vi "Get Edge Mode.vi"(8 "error in (no error)":errorcluster, 11 "VISA resource name":refnum<visa-resource-name>) -> (0 "error out":errorcluster, 2 "Edge Mode":i32, 3 "VISA resource name out":refnum<visa-resource-name>)   [LabVIEW 2013, in "Fluke 5XXX Series Multicalibrators.lvlib"]
doc: "This VI returns the tunnel diode pulse drive setting in the Edge scope mode.\n\nNote:\n\nThis VI is available only for instrument models 5500A and 5520A with oscilloscope option SC600 (SC1100)."
uses:
  Fluke 5XXX Series Multicalibrators.lvlib
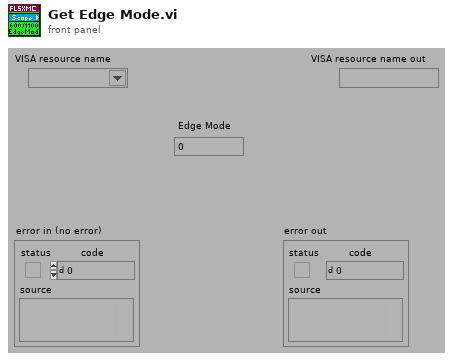
[diagram p1: front panel]
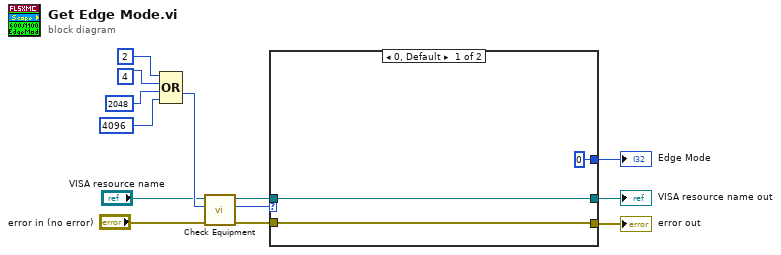
[diagram p0: block diagram]
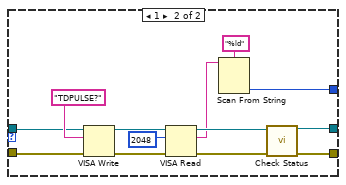
[diagram p2: hidden frame]
diagram:
  n1 = Compound Arithmetic op=OR(2 ("Numeric"), 4 ("Numeric"), 2048 ("Numeric"), 4096 ("Numeric")) -> (w10:i32)
  n2 = call "Check Equipment.vi"("error in (no error)"="error in (no error)", "Bit Mask"=w10, "VISA resource name"="VISA resource name") -> ("error out"=w8:errorcluster, "Present?"=w2:u32, "VISA resource name out"=w7:refnum<visa-resource-name>)  [unwired: 6 in]
  n3 = case shown="0, Default" w2 {
    tunnel: [w16 w23] -> w4
    tunnel: [w15 w20] -> w3
    tunnel: w8 -> [w16 w25]
    tunnel: w7 -> [w15 w24]
    tunnel: [0 w17] -> w1
    frame 0, Default {
    }
    frame 1 {
      n4 = VISA Write(VISA resource name=w24, write buffer="TDPULSE?", error in (no error)=w25) -> (VISA resource name out=w28:refnum<visa-resource-name>, error out=w27:errorcluster)  [unwired: 1 out]
      n5 = VISA Read(VISA resource name=w28, byte count=u32 2048 ("byte count (0)"), error in (no error)=w27) -> (VISA resource name out=w21:refnum<visa-resource-name>, read buffer=w18:string, error out=w22:errorcluster)  [unwired: 1 out]
      n6 = Scan From String(format string="%ld", input string=w18) -> (output 1=w17:i32)  [unwired: 3 in, 3 out]
      n7 = call "Check Status.vi"("VISA resource name"=w21, "error in (no error)"=w22) -> ("VISA resource name out"=w20:refnum<visa-resource-name>, "error out"=w23:errorcluster)  [unwired: 12 in]
    }
  }
  "Edge Mode" <- w1
  "VISA resource name out" <- w3
  "error out" <- w4
